vi "Initialize Coefficients.vi"(8 "error in (no error)":errorcluster, 11 "Servo Drive and  Motor Paras":T1={"Encoder Output Pulses"=900.0, "Gear Ratio(Numerator)"=1000.0, "Gear Ratio(Denominator)"=1.0, "Reduction Ratio"=1.0} {"Gear Ratio(Denominator)" format="%#_10g"}) -> (0 "error out":errorcluster, 1 "Reduction Ratio":dbl, 2 "Enc-Coefficient":dbl, 3 "Vel-Coefficient":dbl)   [LabVIEW 2013, in "SGDV_Ctrl_v13_lib.lvlib"]
uses:
  SGDV_Ctrl_v13_lib.lvlib
  Controls and General VIs/Servo Drive and  Motor Paras.ctl
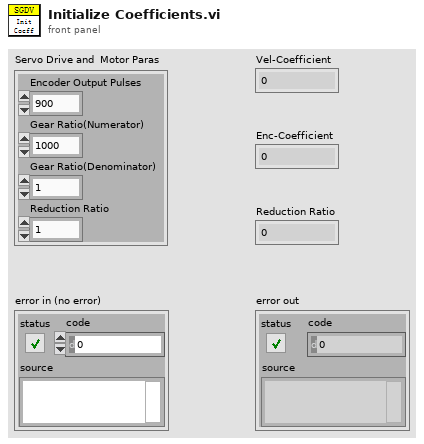
[diagram p1: front panel]
types:
  T1 = typedef "SGDV_Ctrl_v13_lib.lvlib/Servo Drive and  Motor Paras.ctl" = cluster{"Encoder Output Pulses":dbl, "Gear Ratio(Numerator)":dbl, "Gear Ratio(Denominator)":dbl, "Reduction Ratio":dbl}
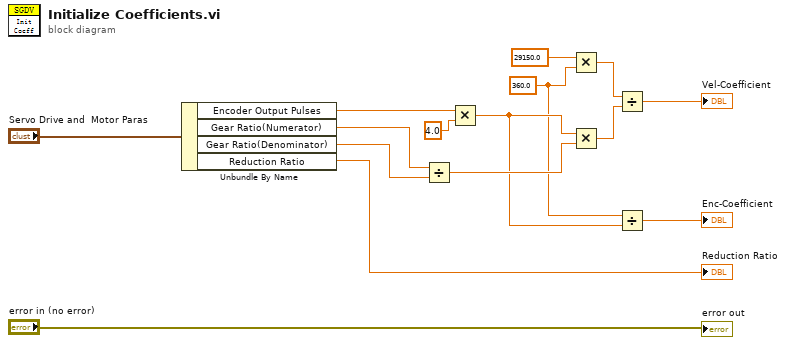
[diagram p0: block diagram]
diagram:
  w7 = 360.0 ("y")
  n1 = Unbundle By Name("Servo Drive and  Motor Paras") -> ("Encoder Output Pulses"=w5:dbl, "Gear Ratio(Numerator)"=w4:dbl, "Gear Ratio(Denominator)"=w3:dbl, "Reduction Ratio"=→"Reduction Ratio":dbl)
  n2 = Divide(x=w4, y=w3) -> (x/y=w10:dbl)
  n3 = Multiply(x=w5, y=4.0) -> (x*y=w8:dbl)
  n4 = Multiply(x=29150.0, y=w7) -> (x*y=w13:dbl)
  n5 = Multiply(x=w8, y=w10) -> (x*y=w12:dbl)
  n6 = Divide(x=w13, y=w12) -> (x/y=→"Vel-Coefficient":dbl)
  n7 = Divide(x=w7, y=w8) -> (x/y=→"Enc-Coefficient":dbl)
  "error out" <- "error in (no error)"
